vi "Global DO.vi"() -> ()   [LabVIEW 2017]
panel:
  in  "HeaterDC":u32
  out "DO":bool[](array[boolean])
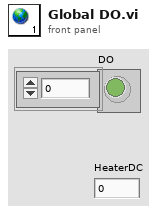
[diagram p1: front panel]
diagram:
